vi "xml_uris.vi"(3 "error in":errorcluster, 5 "Path":path, 6 "Array":T2(array[cluster]) {"duration" step=1}) -> (0 "error out":errorcluster, 1 "String":string, 2 "refnum out":T3)   [LabVIEW 2017]
uses:
  <vilib>/Utility/config.llb/Config Data RefNum.ctl
  Control 1.ctl
  <vilib>/Utility/config.llb/Read Key (String).vi
  <vilib>/Utility/config.llb/NI_LVConfig.lvlib
panel:
  out "standard output 5":string
  out "standard output 4":string
  out "standard output 3":string
  out "standard output 2":string
  out "standard output":string
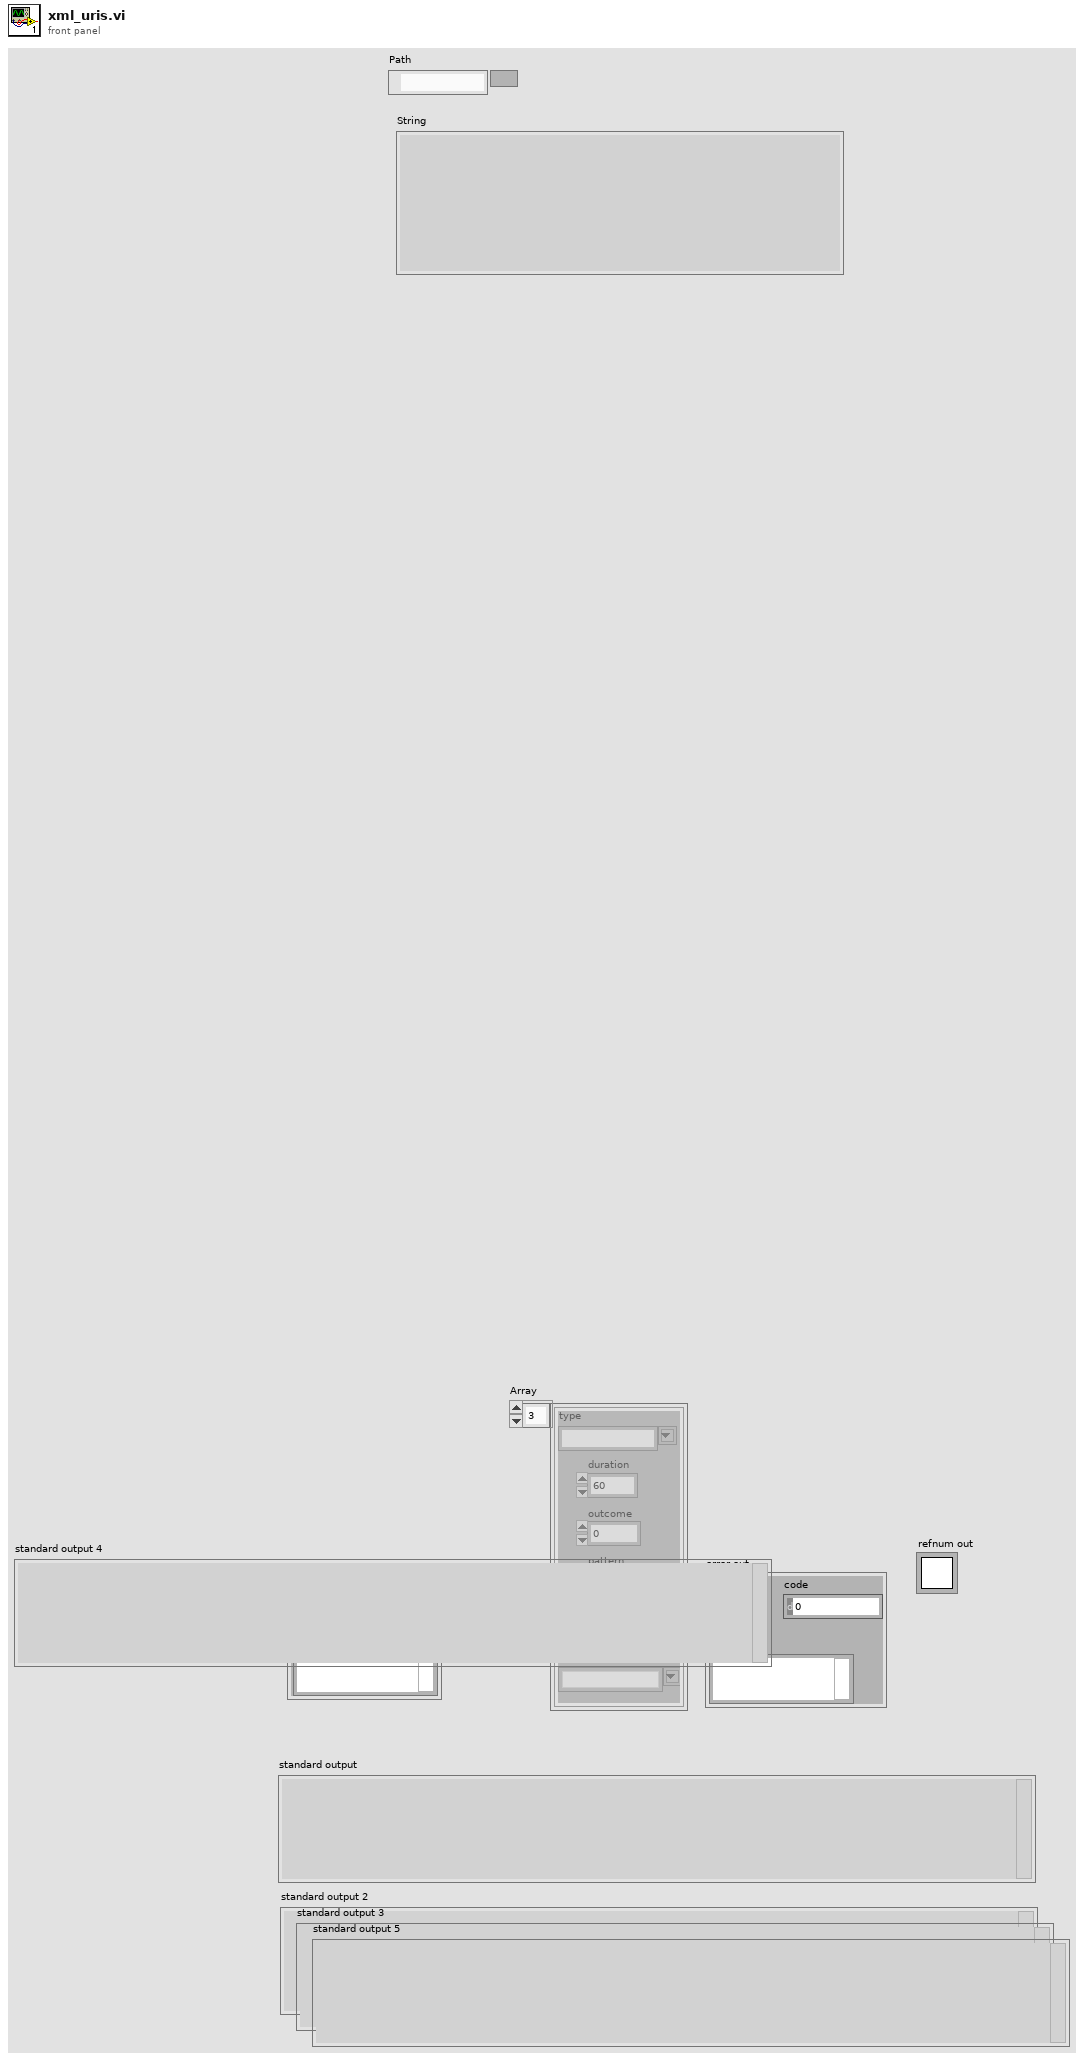
[diagram p1: front panel]
types:
  T1 = typedef "Control 1.ctl" = u32
  T2 = cluster{"type":string, "duration":T1, "outcome":u32, "pattern":u32, "coup_coeff":u32, "contingency":string}[]
  T3 = typedef "NI_LVConfig.lvlib/Config Data RefNum.ctl" = refnum<k1>
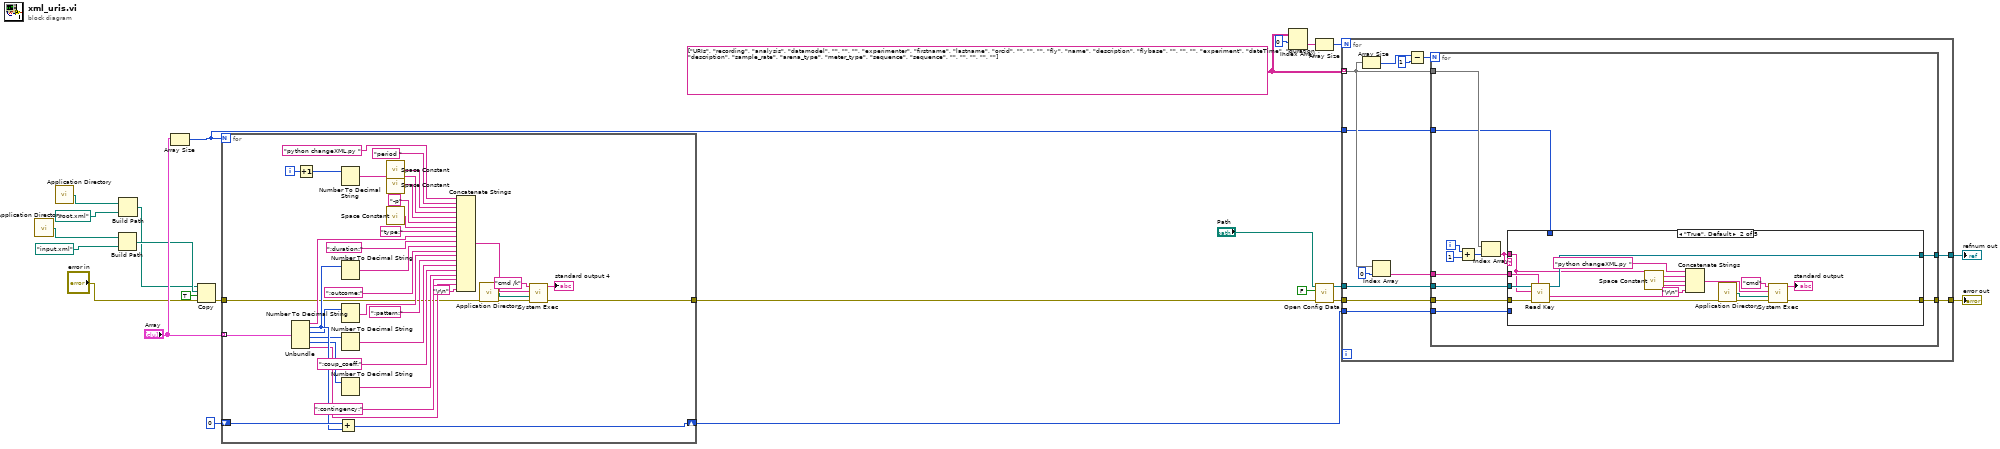
[diagram p0: block diagram]
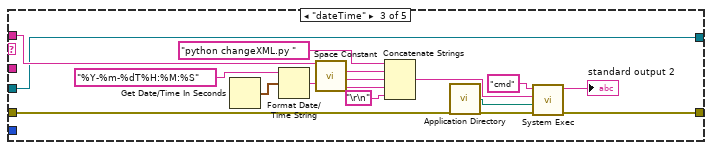
[diagram p3: hidden frame]
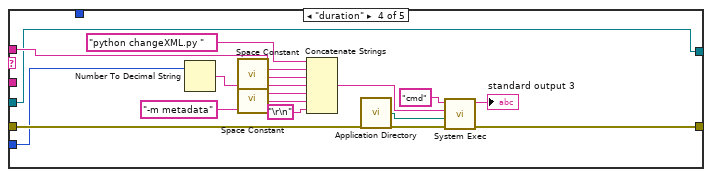
[diagram p4: hidden frame]
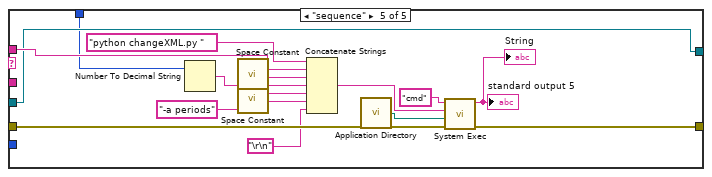
[diagram p5: hidden frame]
diagram:
  w21 = string[][] [["URIs", "recording", "analysis", "datamodel", "", "", ""], ["experimenter", "firstname", "lastname", "orcid", "", "", ""], ["fly", "name", "description", "flybase", "", "", ""], ["experiment", "dateTime", "duration", "description", "sample_rate", "arena_type", "meter_type"], ["sequence", "sequence", "", "", "", "", ""]]
  n1 = call <vilib>:"Application Directory.vi"() -> ("Application Directory"=w6:path)
  n2 = call <vilib>:"Application Directory.vi"() -> ("Application Directory"=w7:path)
  n3 = Build Path(base path=w6, name or relative path=path "input.xml") -> (appended path=w4:path)
  n4 = Build Path(base path=w7, name or relative path=path "root.xml") -> (appended path=w3:path)
  n5 = Array Size(array="Array") -> (size(s)=w2:i32)
  n6 = Copy(8:"error in", 9:TRUE ("overwrite (F)"), 10:w4, 11:w3) -> (0:w11:errorcluster)  [unwired: 1 in, 2 out]
  n7 = for {
    N: w2 -> [_]
    tunnel: "Array" -> [w59] mode=indexing
    shift-right: [w58] -> w13
    shift-left: T1 0 ("duration") -> [w57]
    tunnel: w11 -> [w26]
    tunnel: [w25] -> w12
    i -> [w28]
    n8 = Unbundle(w59) -> ("type"=w44:string, "duration"=w43:T1, "outcome"=w39:u32, "pattern"=w36:u32, "coup_coeff"=w33:u32, "contingency"=w30:string)
    n9 = Increment(x=w28) -> (x+1=w27:i32)
    n10 = Add(x=w57, y=w43) -> (x+y=w58:T1)
    n11 = Number To Decimal String(number=w27) -> (decimal integer string=w50:string)  [unwired: 1 in]
    n12 = Number To Decimal String(number=w43) -> (decimal integer string=w41:string)  [unwired: 1 in]
    n13 = Number To Decimal String(number=w39) -> (decimal integer string=w38:string)  [unwired: 1 in]
    n14 = Number To Decimal String(number=w36) -> (decimal integer string=w35:string)  [unwired: 1 in]
    n15 = Number To Decimal String(number=w33) -> (decimal integer string=w32:string)  [unwired: 1 in]
    n16 = call <vilib>:"Space Constant.vi"() -> ("String"=w53:string)
    n17 = call <vilib>:"Space Constant.vi"() -> ("String"=w48:string)
    n18 = call <vilib>:"Space Constant.vi"() -> ("String"=w46:string)
    n19 = Concatenate Strings("python changeXML.py " ("standard input"), "period " ("string"), w53, w50, w48, "-p" ("string"), w46, "type:" ("string"), w44, ";duration:" ("string"), w41, ";outcome:" ("string"), w38, ";pattern:" ("string"), w35, ";coup_coeff:" ("string"), w32, ";contingency:" ("string"), w30, "\r\n") -> (w52:string)
    n20 = call <vilib>:"Application Directory.vi"() -> ("Application Directory"=w55:path)
    n21 = call <vilib>:"System Exec.vi"("error in (no error)"=w26, "working directory"=w55, "standard input"=w52, "command line"="cmd /k") -> ("error out"=w25:errorcluster, "standard output"=→"standard output 4":string)  [unwired: 4 in, 2 out]
  }
  n22 = Index Array(array=w21, index (row)=0) -> (element=w23:string[])  [unwired: 1 in]
  n23 = Array Size(array=w23) -> (size(s)=w22:i32)
  n24 = call <vilib>:"Open Config Data.vi"("error in (no error)"=w12, "create file if necessary (T)"=FALSE, "configuration file path"="Path") -> ("error out"=w17:errorcluster, "refnum"=w16:T3)  [unwired: 6 in, 1 out]
  n25 = for {
    N: w22 -> [_]
    tunnel: w16 -> [w71]
    tunnel: w21 -> [w70] mode=indexing
    tunnel: w17 -> [w66]
    tunnel: [w65] -> w20
    tunnel: [w62] -> w19
    tunnel: w13 -> [w61]
    tunnel: w2 -> [w60]
    n26 = Array Size(array=w70) -> (size(s)=w68:i32)
    n27 = Index Array(array=w70, index=0) -> (element=w63:string)
    n28 = Subtract(x=w68, y=1) -> (x-y=w69:i32)
    n29 = for {
      N: w69 -> [_]
      tunnel: [w83] -> w62
      tunnel: w71 -> [w82]
      tunnel: w70 -> [w80]
      tunnel: w66 -> [w77]
      tunnel: [w76] -> w65
      tunnel: w63 -> [w75]
      tunnel: w61 -> [w73]
      tunnel: w60 -> [w72]
      i -> [w79]
      n30 = Add(x=w79, y=1) -> (x+y=w78:i32)
      n31 = Index Array(array=w80, index=w78) -> (element=w74:string)
      n32 = case shown="\"True\", Default" w74 {
        tunnel: [w85 w97 w105 w121 w137] -> w83
        tunnel: w82 -> [w85 w98 w105 w121 w137]
        tunnel: w77 -> [w84 w100 w106 w122 w138]
        tunnel: [w84 w95 w104 w120 w136] -> w76
        tunnel: w74 -> [_ w91 w107 w123 w139]
        tunnel: w75 -> [_ w99 _ _ _]
        tunnel: w73 -> [_ _ _ w118 _]
        tunnel: w72 -> [_ _ _ _ w132]
        frame "" {
        }
        frame "True", Default {
          n33 = call-poly <vilib>:"Read Key.vi"("section"=w99, "error in (no error)"=w100, "key"=w91, "refnum"=w98) -> ("error out"=w96:errorcluster, "value"=w90:string, "refnum out"=w97:T3)  [unwired: 4 in, 1 out]
          n34 = call <vilib>:"Space Constant.vi"() -> ("String"=w89:string)
          n35 = Concatenate Strings("python changeXML.py " ("standard input"), w91, w89, w90, "\r\n") -> (w88:string)
          n36 = call <vilib>:"Application Directory.vi"() -> ("Application Directory"=w93:path)
          n37 = call <vilib>:"System Exec.vi"("error in (no error)"=w96, "working directory"=w93, "standard input"=w88, "command line"="cmd") -> ("error out"=w95:errorcluster, "standard output"=→"standard output":string)  [unwired: 4 in, 2 out]
        }
        frame "dateTime" {
          n38 = Get Date/Time In Seconds() -> (seconds since 1Jan1904=w103:timestamp)
          n39 = Format Date/Time String(time format string (%c)="%Y-%m-%dT%H:%M:%S", seconds (now)=w103) -> (date/time string=w101:string)  [unwired: 1 in]
          n40 = call <vilib>:"Space Constant.vi"() -> ("String"=w111:string)
          n41 = Concatenate Strings("python changeXML.py " ("standard input"), w107, w111, w101, "\r\n") -> (w110:string)
          n42 = call <vilib>:"Application Directory.vi"() -> ("Application Directory"=w113:path)
          n43 = call <vilib>:"System Exec.vi"("error in (no error)"=w106, "working directory"=w113, "standard input"=w110, "command line"="cmd") -> ("error out"=w104:errorcluster, "standard output"=→"standard output 2":string)  [unwired: 4 in, 2 out]
        }
        frame "duration" {
          n44 = Number To Decimal String(number=w118) -> (decimal integer string=w119:string)  [unwired: 1 in]
          n45 = call <vilib>:"Space Constant.vi"() -> ("String"=w126:string)
          n46 = call <vilib>:"Space Constant.vi"() -> ("String"=w117:string)
          n47 = Concatenate Strings("python changeXML.py " ("standard input"), w123, w126, w119, w117, "-m metadata" ("string"), "\r\n") -> (w125:string)
          n48 = call <vilib>:"Application Directory.vi"() -> ("Application Directory"=w128:path)
          n49 = call <vilib>:"System Exec.vi"("error in (no error)"=w122, "working directory"=w128, "standard input"=w125, "command line"="cmd") -> ("error out"=w120:errorcluster, "standard output"=→"standard output 3":string)  [unwired: 4 in, 2 out]
        }
        frame "sequence" {
          n50 = Number To Decimal String(number=w132) -> (decimal integer string=w135:string)  [unwired: 1 in]
          n51 = call <vilib>:"Space Constant.vi"() -> ("String"=w141:string)
          n52 = call <vilib>:"Space Constant.vi"() -> ("String"=w134:string)
          n53 = Concatenate Strings("python changeXML.py " ("standard input"), w139, w141, w135, w134, "-a periods" ("string"), "\r\n") -> (w140:string)
          n54 = call <vilib>:"Application Directory.vi"() -> ("Application Directory"=w143:path)
          n55 = call <vilib>:"System Exec.vi"("error in (no error)"=w138, "working directory"=w143, "standard input"=w140, "command line"="cmd") -> ("error out"=w136:errorcluster, "standard output"=→"standard output 5" →"String":string)  [unwired: 4 in, 2 out]
        }
      }
    }
  }
  "error out" <- w20
  "refnum out" <- w19
